vi "Write INI File.vi"(8 "error in":errorcluster, 10 "File path":T1, 11 "INI refnum":T2) -> (0 "error out":errorcluster)   [LabVIEW 2025, in "Config Tool.lvlib"]
uses:
  Config Tool.lvlib
  <vilib>/Utility/config.llb/Config Data RefNum.ctl
  Controls/FilePaths.ctl
  <vilib>/Utility/config.llb/Write Key (Path).vi
  <vilib>/Utility/config.llb/NI_LVConfig.lvlib
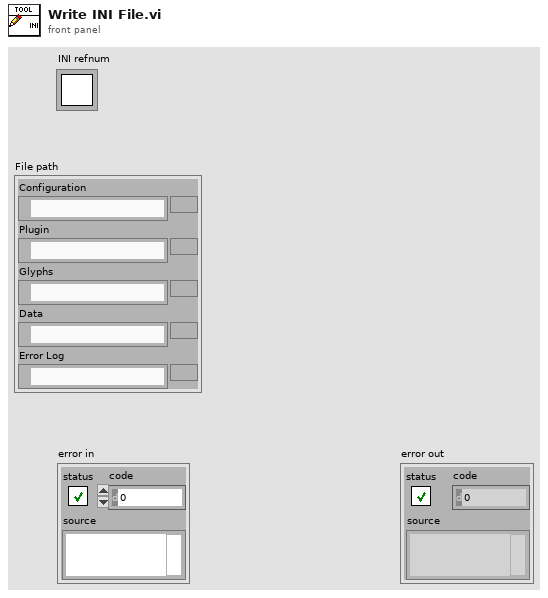
[diagram p1: front panel]
types:
  T1 = typedef "Config Tool.lvlib/FilePaths.ctl" = cluster{"Configuration":path, "Plugin":path, "Glyphs":path, "Data":path, "Error Log":path}
  T2 = typedef "NI_LVConfig.lvlib/Config Data RefNum.ctl" = refnum<k1>
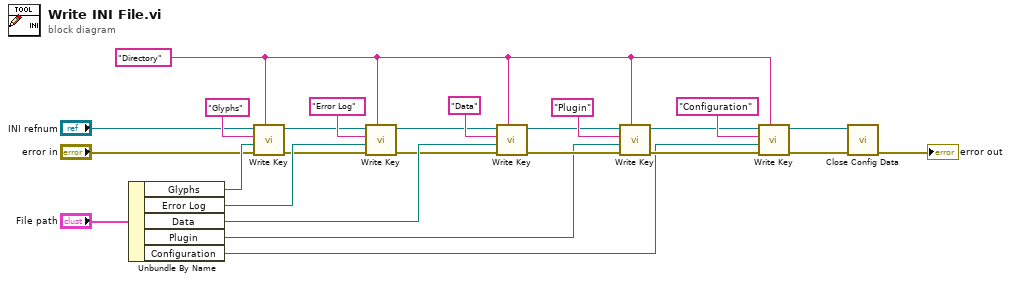
[diagram p0: block diagram]
diagram:
  w9 = "Directory" ("section")
  n1 = Unbundle By Name("File path") -> ("Glyphs"=w5:path, "Error Log"=w6:path, "Data"=w12:path, "Plugin"=w13:path, "Configuration"=w14:path)
  n2 = call-poly <vilib>:"Write Key.vi"("section"=w9, "error in (no error)"="error in", "value"=w5, "key"="Glyphs", "refnum"="INI refnum") -> ("error out"=w2:errorcluster, "refnum out"=w8:T2)  [unwired: 4 in, 1 out]
  n3 = call-poly <vilib>:"Write Key.vi"("section"=w9, "error in (no error)"=w2, "value"=w6, "key"="Error Log", "refnum"=w8) -> ("error out"=w3:errorcluster, "refnum out"=w7:T2)  [unwired: 4 in, 1 out]
  n4 = call-poly <vilib>:"Write Key.vi"("section"=w9, "error in (no error)"=w3, "value"=w12, "key"="Data", "refnum"=w7) -> ("error out"=w16:errorcluster, "refnum out"=w17:T2)  [unwired: 4 in, 1 out]
  n5 = call-poly <vilib>:"Write Key.vi"("section"=w9, "error in (no error)"=w16, "value"=w13, "key"="Plugin", "refnum"=w17) -> ("error out"=w23:errorcluster, "refnum out"=w22:T2)  [unwired: 4 in, 1 out]
  n6 = call-poly <vilib>:"Write Key.vi"("section"=w9, "error in (no error)"=w23, "value"=w14, "key"="Configuration", "refnum"=w22) -> ("error out"=w19:errorcluster, "refnum out"=w20:T2)  [unwired: 4 in, 1 out]
  n7 = call <vilib>:"Close Config Data.vi"("error in (no error)"=w19, "refnum"=w20) -> ("error out"=→"error out":errorcluster)  [unwired: 8 in, 1 out]
